vi "json Insert Variant - string path.vi"(8 "error in (no error)":errorcluster, 9 "anything":variant, 10 "path":string, 11 "JSON Document in":refnum<class "JSON Document.lvclass">) -> (0 "error out":errorcluster, 1 "replaced?":bool, 3 "JSON Document out":refnum<class "JSON Document.lvclass">)   [LabVIEW 2015, in "JSON Document.lvclass"]
uses:
  JSON Document.lvclass
  JSON Document.lvclass/JSON Document.ctl
  rapidjson wrapper/rapidjson wrapper.lvlib
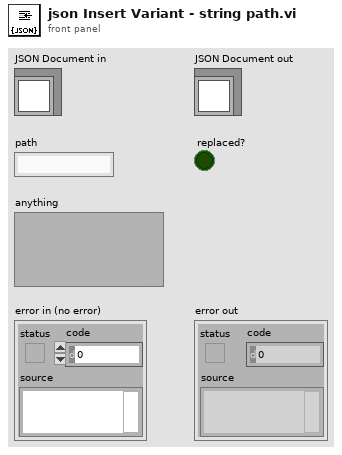
[diagram p1: front panel]
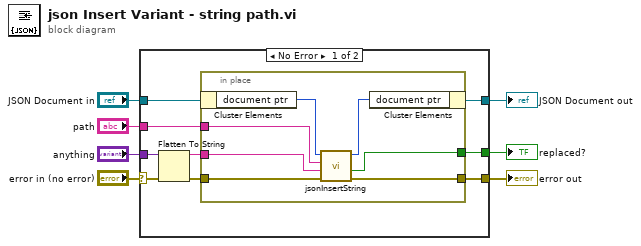
[diagram p0: block diagram]
diagram:
  n1 = case shown="No Error" "error in (no error)" {
    selector: "error in (no error)" -> [w11 w25]
    tunnel: [w13 w25] -> w6
    tunnel: [w15 w24] -> w4
    tunnel: "JSON Document in" -> [w16 w24]
    tunnel: "anything" -> [w12 _]
    tunnel: "path" -> [w14 _]
    tunnel: [w8 _] -> w1
    frame No Error {
      n2 = Flatten To String(anything=w12, error in (no error)=w11) -> (data string=w9:string, error out=w10:errorcluster)  [unwired: 2 in, 1 out]
      n3 = in-place {
        in-place-border: w14 -> [w18]
        in-place-border: w10 -> [w22]
        in-place-border: [w20] -> w13
        in-place-border: w9 -> [w21]
        in-place-border: [w17] -> w8
        n4 = in-place-cluster #1(w16) -> ("document ptr"=w19:i64)
        n5 = call "jsonInsertString.vi"("error in (no error)"=w22, "value"=w21, "path"=w18, "d in"=w19) -> ("error out"=w20:errorcluster, "replaced?"=w17:bool, "d out"=w23:i64)  [unwired: 5 in]
        n6 = in-place-cluster #1("document ptr"=w23) -> (w15:refnum<class "JSON Document.lvclass">)
      }
    }
    frame Error {
    }
  }
  "error out" <- w6
  "JSON Document out" <- w4
  "replaced?" <- w1
